vi "Stop or Error.vi"(8 "error in (no error)":errorcluster, 9 "stop":bool) -> (0 "error out":errorcluster, 1 "Shutdown?":bool)   [LabVIEW 2012]
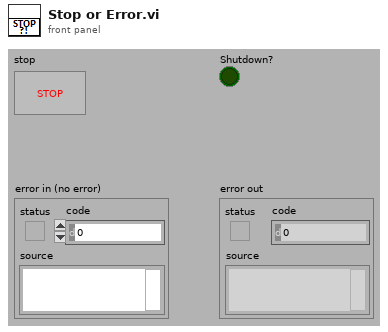
[diagram p1: front panel]
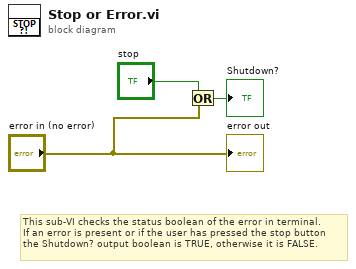
[diagram p0: block diagram]
diagram:
  # "This sub-VI checks the status boolean of the error in terminal.\nIf an error is present or if the user has pressed the stop button\nthe Shutdown? output boolean is TRUE, otherwise it is FALSE."
  n1 = Or(x="stop", y="error in (no error)") -> (x .or. y?=→"Shutdown?":bool)
  "error out" <- "error in (no error)"
